vi "Initialize Events.vi"(8 "Error in":errorcluster caption="Error in (no error)") -> (0 "Error out":errorcluster, 3 "Editor Events":T1)   [LabVIEW 2023, in "VIDocEditor.lvclass"]
uses:
  VIDocEditor.lvclass
  Editor Events Cluster.ctl
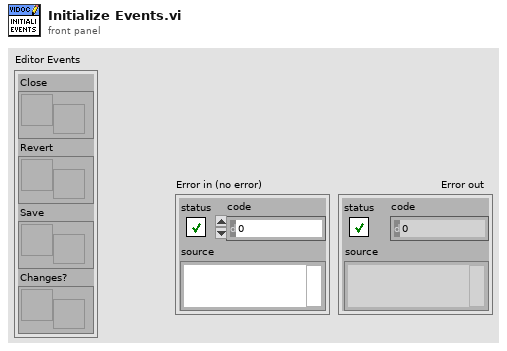
[diagram p1: front panel]
types:
  T1 = typedef "VIDocEditor.lvclass/Editor Events Cluster.ctl" = cluster{"Close":refnum<user-event>, "Revert":refnum<user-event>, "Save":refnum<user-event>, "Changes?":refnum<user-event>}
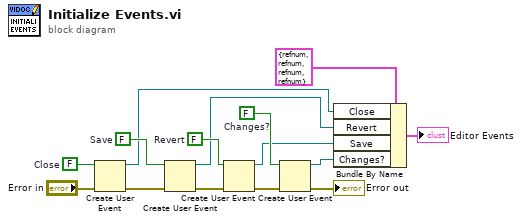
[diagram p0: block diagram]
diagram:
  w12 = FALSE  # Changes?
  w13 = FALSE  # Revert
  w14 = FALSE  # Save
  w15 = FALSE  # Close
  n1 = Create User Event(user event datatype=w15, error in="Error in") -> (user event=w4:refnum<user-event>, error out=w10:errorcluster)
  n2 = Create User Event(user event datatype=w14, error in=w10) -> (user event=w3:refnum<user-event>, error out=w9:errorcluster)
  n3 = Create User Event(user event datatype=w13, error in=w9) -> (user event=w2:refnum<user-event>, error out=w8:errorcluster)
  n4 = Create User Event(user event datatype=w12, error in=w8) -> (user event=w1:refnum<user-event>, error out=→"Error out":errorcluster)
  n5 = Bundle By Name(cluster=T1 {"Close"=refnum, "Revert"=refnum, "Save"=refnum, "Changes?"=refnum} ("Editor Events"), "Close"=w4, "Revert"=w3, "Save"=w2, "Changes?"=w1) -> (→"Editor Events":T1)
